vi "DataWriteTxtGen.vi"(0 "DataFileRef":refnum<file>, 5 "LastScanPosIn":dbl, 9 "NewYDataIn":dbl[](array[numeric]) format="%#_16g", 11 "error in (no error)":errorcluster) -> (4 "DataFileRef Out":refnum<file>, 6 "LastScanPosOut":dbl, 10 "NewYDataOut":dbl[](array[numeric]), 15 "error out":errorcluster)   [LabVIEW 2010]
doc: "Ce VI sauvegarde les données d'acquisition pour en garder une copie de sécurité qui peut être rappeller en cas de panne."
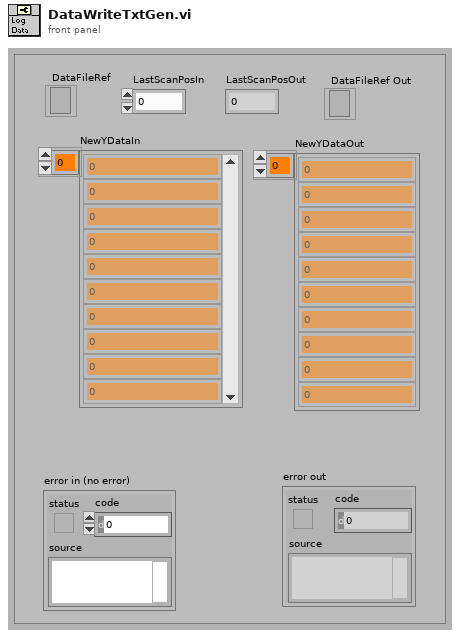
[diagram p1: front panel]
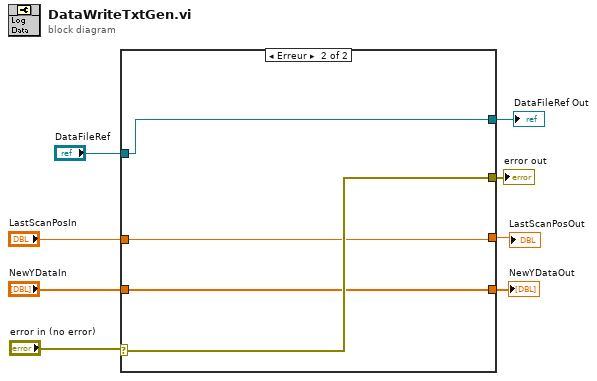
[diagram p0: block diagram]
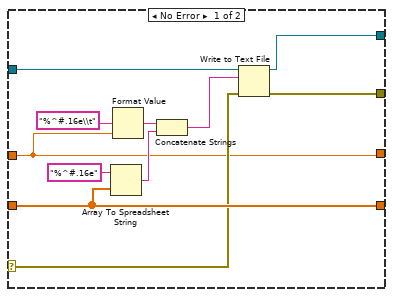
[diagram p2: hidden frame]
diagram:
  n1 = case shown="Erreur" "error in (no error)" {
    selector: "error in (no error)" -> [w11 w23]
    tunnel: "LastScanPosIn" -> [w10 w21]
    tunnel: "NewYDataIn" -> [w19 w22]
    tunnel: [w13 w23] -> w5
    tunnel: [w19 w22] -> w4
    tunnel: "DataFileRef" -> [w12 w20]
    tunnel: [w10 w21] -> w2
    tunnel: [w9 w20] -> w1
    frame No Error {
      n2 = Array To Spreadsheet String(array=w19, 3:"%^#.16e" ("chaîne de format")) -> (spreadsheet string=w15:string)  [unwired: 1 in]
      n3 = Format Value(format string="%^#.16e\\t" ("chaîne de format"), value (0)=w10) -> (output string=w16:string)  [unwired: 1 in]
      n4 = Concatenate Strings(w16, w15) -> (w14:string)
      n5 = Write to Text File(file (use dialog)=w12, text=w14, error in=w11) -> (refnum out=w9:refnum<file>, error out=w13:errorcluster)  [unwired: 1 in, 1 out]
    }
    frame Error {
    }
  }
  "NewYDataOut" <- w4
  "error out" <- w5
  "LastScanPosOut" <- w2
  "DataFileRef Out" <- w1
